vi "gXOR_gt_nand.vi"() -> ()   [LabVIEW 2026]
panel:
  out "Boolean 3":bool
  in  "Boolean 2":bool
  in  "Boolean":bool
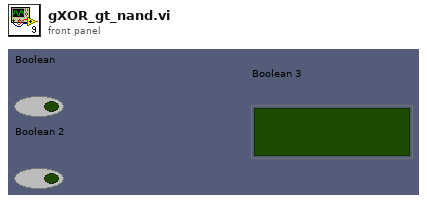
[diagram p1: front panel]
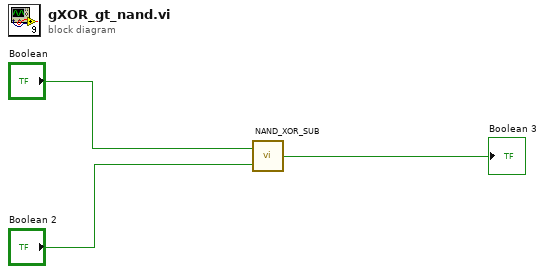
[diagram p0: block diagram]
diagram:
  n1 = call "NAND_XOR_SUB.vi"("Boolean 2"="Boolean 2", "Boolean"="Boolean") -> ("Boolean 3"=→"Boolean 3":bool)
